vi "GV-CursorZoomwindowStart.vi"(6 "Y":dbl, 7 "Gviewer in":refnum<class "Gviewer.lvclass">, 8 "error in (no error)":errorcluster, 10 "Pos":cluster{"x":i16, "y":i16}, 11 "pict in":picture) -> (0 "error out":errorcluster, 3 "pict out":picture)   [LabVIEW 2020, in "Sgraph_lib_V1.lvlib" / "Gviewer.lvclass"]
doc: "Andre Koelewijn, 2 may 2021\n\nDefine starting point for Windowed Zoom.\nThis function allows zooming for one selected TAG or all TAGs"
uses:
  Gviewer.lvclass
  Gviewer.lvclass/Gviewer.ctl
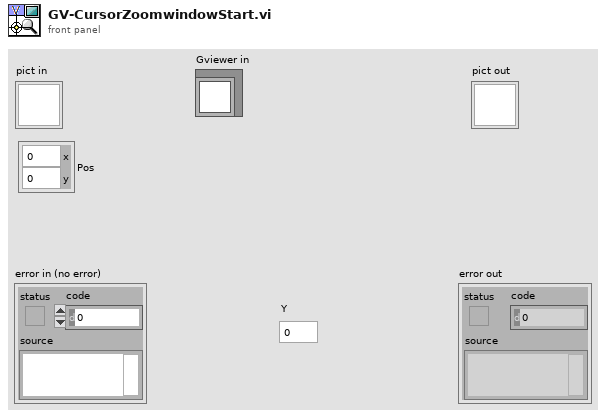
[diagram p1: front panel]
types:
  T1 = cluster{"horizontal":enum16{"left", "center", "right"}, "vertical":enum16{"top", "center", "bottom"}}
  T2 = cluster{"Width":u16, "Style":enum32{"Solid", "Dash", "Dot", "DashDot", "DashDotDot"}}
  T3 = typedef "Sgraph_lib_V1.lvlib/Gviewer.lvclass/Typedef_SelProperties.ctl" = cluster{"Color":u32, "LineType":T4, "max":dbl, "min":dbl}
  T4 = typedef "Sgraph_lib_V1.lvlib/Gviewer.lvclass/Typedef_LineType.ctl" = enum16{"num_bare", "num_MinMax_Area", "num_MinMax_Lines", "num_MinMax_Forfor", "num_Max_Area", "num_Max_Line", "num_Max_Forfor", "num_Min_Area", "num_Min_Line", "num_Min_Fosfor", "Boolean_Line_01", "Boolean_Area_01", "Boolean_Fosfor_01", "Boolean_Line_TF", "Boolean_Area_TF", "Boolean_Fosfor_TF", "Boolean_OnOff_Line", "Boolean_OnOff_Area", "Boolean_OnOff_Fosfor", "Boolean_spare", "StringEvent_Line", "StringEvent_TimeLine"}
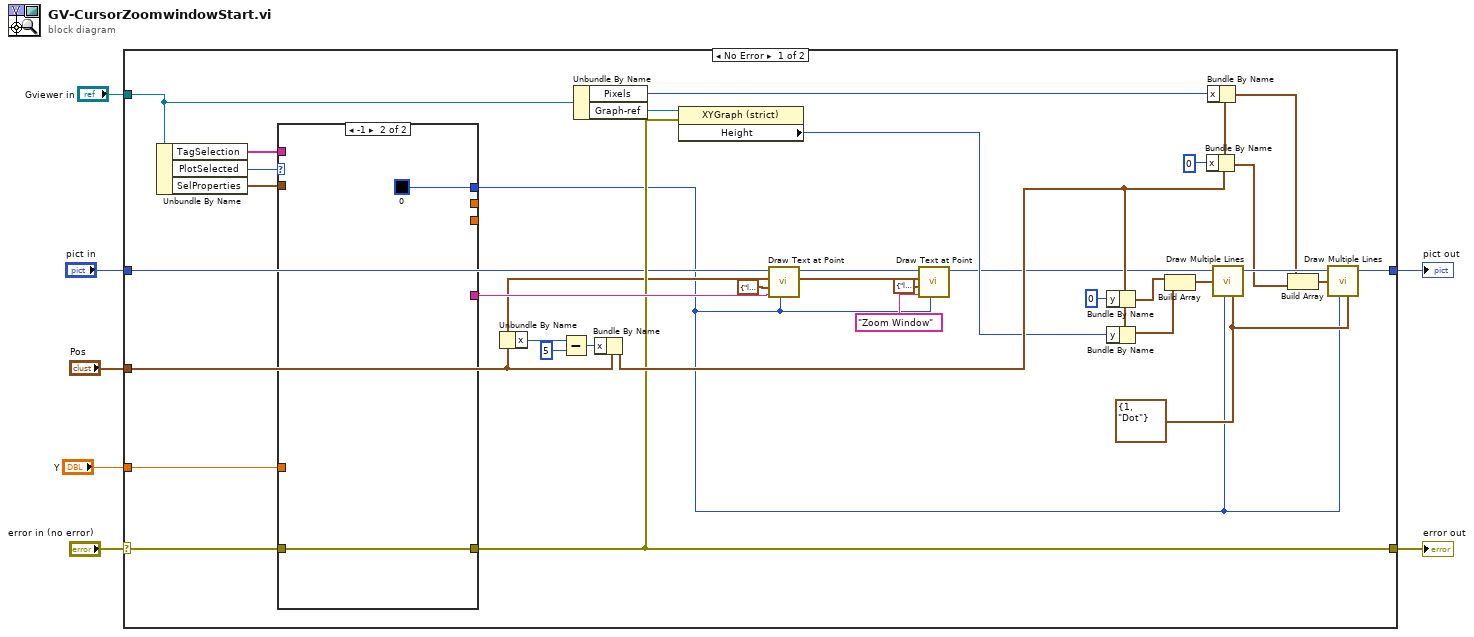
[diagram p0: block diagram]
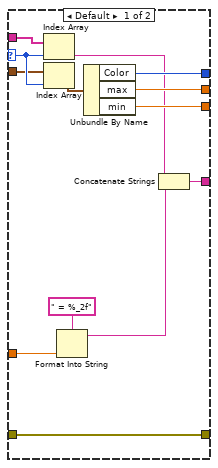
[diagram p2: hidden frame]
diagram:
  n1 = case shown="No Error" "error in (no error)" {
    selector: "error in (no error)" -> [w21 w59]
    tunnel: [w14 w59] -> w6
    tunnel: "pict in" -> [w11 w58]
    tunnel: [w36 w58] -> w4
    tunnel: "Pos" -> [w12 _]
    tunnel: "Gviewer in" -> [w26 _]
    tunnel: "Y" -> [w19 _]
    frame No Error {
      w18 = T2 {"Width"=1, "Style"=enum."Dot"} ("pen")
      n2 = Unbundle By Name(w26) -> ("TagSelection"=w28:string[], "PlotSelected"=w20:i32, "SelProperties"=w30:T3[])
      n3 = case shown="-1" w20 {
        selector: w20 -> [w51 _]
        tunnel: w28 -> [w54 _]
        tunnel: [w47 "All TAGs"] -> w29
        tunnel: w30 -> [w46 _]
        tunnel: [w52 u32 0 ("Color")] -> w8
        tunnel: [w50 _] -> _
        tunnel: [w49 _] -> _
        tunnel: w21 -> [w43 w55]
        tunnel: [w43 w55] -> w14
        tunnel: w19 -> [w42 _]
        frame Default {
          n4 = Index Array(array=w54, index=w51) -> (element=w48:string)
          n5 = Index Array(array=w46, index=w51) -> (element=w53:T3)
          n6 = Format Into String(format string=" = %_2f", w42) -> (resulting string=w44:string)  [unwired: 2 in, 1 out]
          n7 = Unbundle By Name(w53) -> ("Color"=w52:u32, "max"=w50:dbl, "min"=w49:dbl)
          n8 = Concatenate Strings(w48, w44) -> (w47:string)
        }
        frame -1 {
        }
      }
      n9 = Unbundle By Name(w12) -> ("x"=w24:i16)
      n10 = Subtract(x=w24, y=i16 5) -> (x-y=w22:i16)
      n11 = Unbundle By Name(w26) -> ("Pixels"=w25:i32, "Graph-ref"=w15:refnum<vi>)
      n12 = Bundle By Name(cluster=w12, "x"=w22) -> (w16:cluster{"x":i16, "y":i16})
      n13 = property class="XYGraph (strict)"(reference=w15, error in=w14) -> ("Height"=w13:u32)  [unwired: 2 out]
      n14 = call <vilib>:"Draw Text at Point.vi"("text color(black)"=w8, "text"=w29, "alignment(left, top)"=T1 {"horizontal"=enum."left", "vertical"=enum."top"}, "origin"=w12, "picture"=w11) -> ("new picture"=w10:picture)  [unwired: 5 in, 1 out]
      n15 = call <vilib>:"Draw Text at Point.vi"("text color(black)"=w8, "text"="Zoom Window", "alignment(left, top)"=T1 {"horizontal"=enum."left", "vertical"=enum."bottom"}, "origin"=w12, "picture"=w10) -> ("new picture"=w9:picture)  [unwired: 5 in, 1 out]
      n16 = Bundle By Name(cluster=w16, "y"=i16 0 ("x")) -> (w38:cluster{"x":i16, "y":i16})
      n17 = Bundle By Name(cluster=w16, "y"=w13) -> (w40:cluster{"x":i16, "y":i16})
      n18 = Build Array(w38, w40) -> (w41:cluster{"x":i16, "y":i16}[])
      n19 = Bundle By Name(cluster=w16, "x"=i16 0) -> (w34:cluster{"x":i16, "y":i16})
      n20 = Bundle By Name(cluster=w16, "x"=w25) -> (w33:cluster{"x":i16, "y":i16})
      n21 = call <vilib>:"Draw Multiple Lines.vi"("picture"=w9, "line endpoints"=w41, "color(black)"=w8, "pen"=w18) -> ("new picture"=w37:picture)  [unwired: 5 in]
      n22 = Build Array(w33, w34) -> (w35:cluster{"x":i16, "y":i16}[])
      n23 = call <vilib>:"Draw Multiple Lines.vi"("picture"=w37, "line endpoints"=w35, "color(black)"=w8, "pen"=w18) -> ("new picture"=w36:picture)  [unwired: 5 in]
    }
    frame Error {
    }
  }
  "error out" <- w6
  "pict out" <- w4
